vi "00_global_variables.vi"() -> ()   [LabVIEW 2025]
panel:
  in  "plot_y_axis_relation":T1(array[cluster])=[{"y_scale_id"=0, "unit"="db", "prefix_enable"=FALSE, "plot_id"=0}, {"y_scale_id"=1, "unit"="°", "prefix_enable"=FALSE, "plot_id"=1}, {"y_scale_id"=2, "unit"="", "prefix_enable"=FALSE, "plot_id"=2}, {"y_scale_id"=3, "unit"="", "prefix_enable"=FALSE, "plot_id"=3}, {"y_scale_id"=3, "unit"="", "prefix_enable"=FALSE, "plot_id"=4}, {"y_scale_id"=4, "unit"="Ohm", "prefix_enable"=TRUE, "plot_id"=5}, {"y_scale_id"=5, "unit"="Ohm", "prefix_enable"=TRUE, "plot_id"=6}, {"y_scale_id"=4, "unit"="Ohm", "prefix_enable"=TRUE, "plot_id"=7}, {"y_scale_id"=5, "unit"="Ohm", "prefix_enable"=TRUE, "plot_id"=8}, {"y_scale_id"=4, "unit"="Ohm", "prefix_enable"=TRUE, "plot_id"=9}, {"y_scale_id"=6, "unit"="H", "prefix_enable"=TRUE, "plot_id"=10}, {"y_scale_id"=7, "unit"="F", "prefix_enable"=TRUE, "plot_id"=11}, {"y_scale_id"=6, "unit"="H", "prefix_enable"=TRUE, "plot_id"=12}, {"y_scale_id"=7, "unit"="F", "prefix_enable"=TRUE, "plot_id"=13}, {"y_scale_id"=0, "unit"="db", "prefix_enable"=FALSE, "plot_id"=14}, {"y_scale_id"=1, "unit"="°", "prefix_enable"=FALSE, "plot_id"=15}, {"y_scale_id"=8, "unit"="s", "prefix_enable"=TRUE, "plot_id"=16}, {"y_scale_id"=3, "unit"="", "prefix_enable"=FALSE, "plot_id"=17}, {"y_scale_id"=3, "unit"="", "prefix_enable"=FALSE, "plot_id"=18}, {"y_scale_id"=9, "unit"="%", "prefix_enable"=FALSE, "plot_id"=19}, {"y_scale_id"=9, "unit"="%", "prefix_enable"=FALSE, "plot_id"=20}, {"y_scale_id"=9, "unit"="%", "prefix_enable"=FALSE, "plot_id"=21}]
  # "Y-Scale ID in Graph (Should be everywhere the same)"
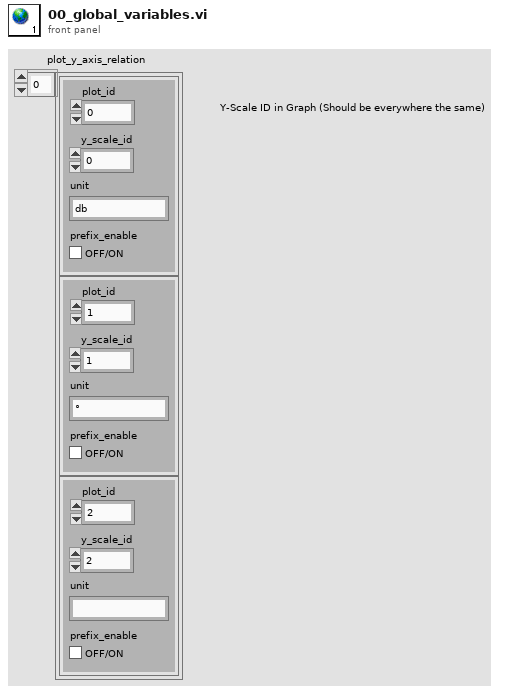
[diagram p1: front panel]
types:
  T1 = cluster{"y_scale_id":u32, "unit":string, "prefix_enable":bool, "plot_id":u32}[]
diagram:
